vi "Evaluate Meta Data.vi"(8 "error IO":errorcluster, 11 "Plugin_Controller":refnum<class "Plugin_Controller.lvclass">) -> (0 "error out":errorcluster, 3 "Device Meta Data":T1)   [LabVIEW 2020, in "Plugin.lvlib" / "Plugin_UI.lvclass"]
doc: "Read Device meta data from Distributor"
uses:
  Plugin_UI.lvclass
  builds/Libraries/Shared GUI Library.lvlibp/Shared GUI Library/Device Meta Data Cluster/DeviceMetaDataCluster.ctl
  builds/Libraries/design.lvlibp/GUI/Design/CustomButtons/LineType/clear_list_l.ctl
  Controller_Class/Plugin_Controller.lvclass
  C:/SVN_LabSys/labsys_lvcode/LabSys_SourceCode/builds/Libraries/LabSys Framework.lvlibp/Data Node/Data Node/Data Node.lvclass
  C:/SVN_LabSys/labsys_lvcode/LabSys_SourceCode/builds/Libraries/LabSys Framework.lvlibp/Configurable Data Node/Configurable Data Node/Configurable Data Node.lvclass
  builds/Libraries/LabSys Framework.lvlibp/Node Meta Data Distributor/Node Meta Data Distributor/Node Meta Data Distributor.lvclass
  builds/Libraries/LabSys Framework.lvlibp/Configuration Storage/Test Configuration/Test Configuration.lvclass
  builds/Libraries/LabSys Framework.lvlibp/Data Node/Data Node/Read Node Meta Data Distributor.vi
  builds/Libraries/LabSys Framework.lvlibp/Data Node/Data Node/Read Module Name.vi
  builds/Libraries/LabSys Framework.lvlibp/Configurable Data Node/Configurable Data Node/Read Module Configuration.vi
  builds/Libraries/LabSys Framework.lvlibp/Configuration Storage/Module Configuration/Module Configuration.lvclass
  builds/Libraries/design.lvlibp
  builds/Libraries/Shared GUI Library.lvlibp
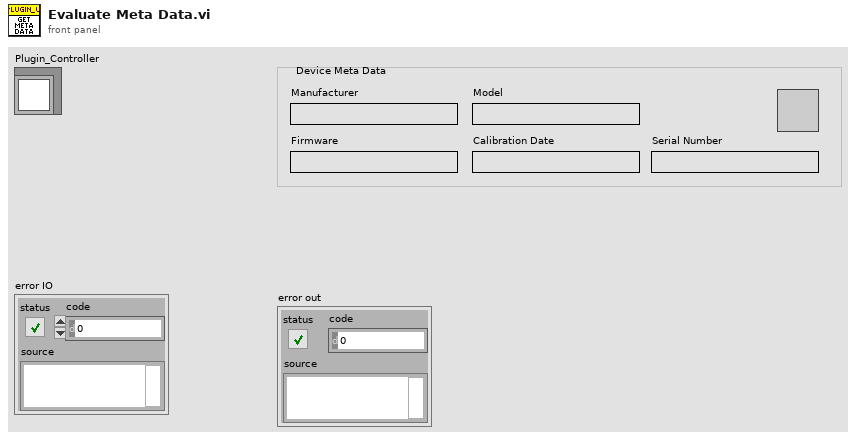
[diagram p1: front panel]
types:
  T1 = typedef "Shared GUI Library.lvlibp/DeviceMetaDataCluster.ctl" = cluster{"Manufacturer":string, "Model":string, "Serial Number":string, "Firmware":string, "Calibration Date":string, "Refresh":T2}
  T2 = typedef "design.lvlibp/clear_list_l.ctl" = bool
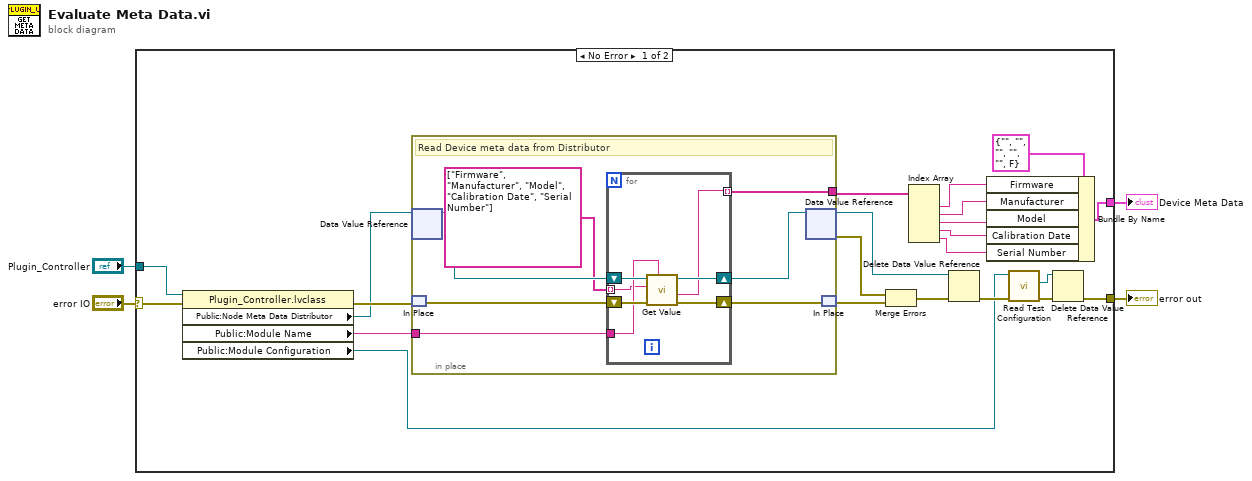
[diagram p0: block diagram]
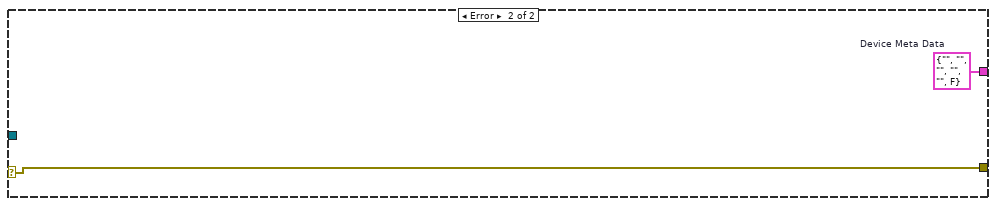
[diagram p2: hidden frame]
diagram:
  n1 = case shown="No Error" "error IO" {
    selector: "error IO" -> [w7 w42]
    tunnel: "Plugin_Controller" -> [w21 _]
    tunnel: [w15 w42] -> w2
    tunnel: [w8 w41] -> w3
    frame No Error {
      n2 = property class="Plugin_Controller.lvclass"(reference=w21, error in=w7) -> (error out=w23:errorcluster, "Public:Node Meta Data Distributor"=w22:refnum<data-value>, "Public:Module Name"=w24:string, "Public:Module Configuration"=w14:refnum<class "Module Configuration.lvclass">)  [unwired: 1 out]
      n3 = in-place {
        in-place-border: w24 -> [w29]
        in-place-border: [w27] -> w12
        # "Read Device meta data from Distributor"
        n4 = in-place-dvr #1(w22) -> (w33:refnum<class "Node Meta Data Distributor.lvclass">)  [unwired: 1 out]
        n5 = in-place-match #2(w23) -> (w31:errorcluster)
        n6 = for {
          tunnel: w29 -> [w37]
          shift-right: [w39] -> w32
          shift-left: w33 -> [w40]
          shift-right: [w35] -> w30
          shift-left: w31 -> [w38]
          tunnel: string[] ["Firmware", "Manufacturer", "Model", "Calibration Date", "Serial Number"] -> [w36] mode=indexing
          tunnel: [w34] -> w27 mode=indexing
          n7 = call "Get Value.vi"("Module Name"=w37, "error in (no error)"=w38, "Key"=w36, "Node Meta Data Distributor in"=w40) -> ("error out"=w35:errorcluster, "Value"=w34:string, "Node Meta Data Distributor out"=w39:refnum<class "Node Meta Data Distributor.lvclass">)  [unwired: 4 in, 1 out]
        }
        n8 = in-place-dvr #1(w32) -> (w19:refnum<data-value>, w26:errorcluster)
        n9 = in-place-match #2(w30) -> (w25:errorcluster)
      }
      n10 = Merge Errors(w26, w25) -> (w20:errorcluster)
      n11 = Index Array(array=w12) -> (element #1=w11:string, element #2=w10:string, element #3=w9:string, element #4=w6:string, element #5=w5:string)  [unwired: 5 in]
      n12 = Delete Data Value Reference(data value reference=w19, error in=w20) -> (error out=w16:errorcluster)  [unwired: 1 out]
      n13 = Bundle By Name(cluster=T1 {"Manufacturer"="", "Model"="", "Serial Number"="", "Firmware"="", "Calibration Date"="", "Refresh"=FALSE} ("Device Meta Data"), "Firmware"=w11, "Manufacturer"=w10, "Model"=w9, "Calibration Date"=w6, "Serial Number"=w5) -> (w8:T1)
      n14 = call "Read Test Configuration.vi"("error in (no error)"=w16, "Module Configuration in"=w14) -> ("error out"=w17:errorcluster, "Test Configuration"=w18:refnum<data-value>)  [unwired: 7 in, 1 out]
      n15 = Delete Data Value Reference(data value reference=w18, error in=w17) -> (error out=w15:errorcluster)  [unwired: 1 out]
    }
    frame Error {
      w41 = T1 {"Manufacturer"="", "Model"="", "Serial Number"="", "Firmware"="", "Calibration Date"="", "Refresh"=FALSE}  # Device Meta Data
    }
  }
  "Device Meta Data" <- w3
  "error out" <- w2
